vi "case.vi"() -> ()   [LabVIEW 2017]
panel:
  out "Title case":string
  out "start case":string
  out "all lower case string":string
  out "all upper case string":string
  in  "input":string
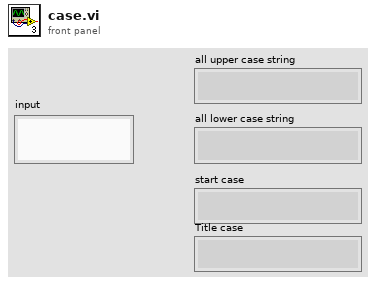
[diagram p1: front panel]
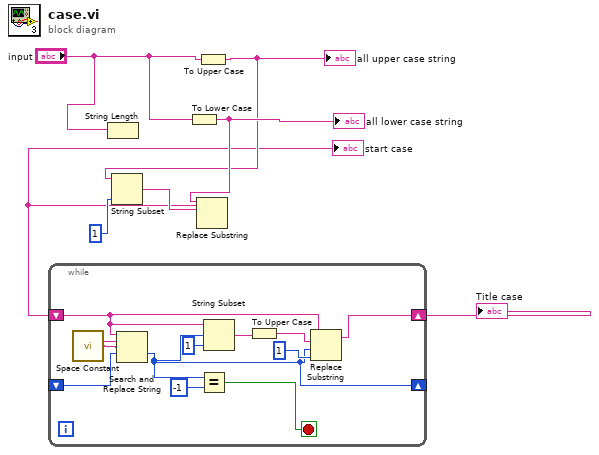
[diagram p0: block diagram]
diagram:
  n1 = String Length(string="input") -> ()  [unwired: 1 out]
  n2 = To Lower Case(string="input") -> (all lower case string=w4:string)
  "all lower case string" <- w4
  n3 = To Upper Case(1:"input") -> (0:w3:string)
  "all upper case string" <- w3
  n4 = String Subset(string=w3, length (rest)=1 ("length (rest)")) -> (substring=w5:string)  [unwired: 1 in]
  n5 = Replace Substring(4:w5, 5:w4) -> (1:w2:string)  [unwired: 2 in, 1 out]
  "start case" <- w2
  n6 = while {
    shift-right: [w11] -> w1
    shift-left: w2 -> [w13]
    shift-right: [w9] -> _
    shift-left: _ -> [w10]
    stop <- w17 stop-if-true
    n7 = call <vilib>:"Space Constant.vi"() -> ("String"=w8:string)
    n8 = Search and Replace String(input string=w13, search string=w8, replace string=w8, offset=w10) -> (offset past replacement=w9:i32)  [unwired: 4 in, 3 out]
    n9 = Equal?(x=w9, y=-1) -> (x = y?=w17:bool)
    n10 = String Subset(string=w13, offset (0)=w9, length (rest)=1 ("length (rest)")) -> (substring=w15:string)
    n11 = To Upper Case(1:w15) -> (0:w14:string)
    n12 = Replace Substring(2:1 ("length (len. of substring)"), 3:w9, 4:w14, 5:w13) -> (1:w11:string)  [unwired: 1 out]
  }
  "Title case" <- w1
